vi "Chrg_Dschrg_2.vi"(3 "Strain Offset":dbl, 4 "PS VISA in":refnum<visa-resource-name>, 5 "PS error in":errorcluster caption="PS error in (no error)", 6 "CyclePath":path=path "C:/Users/ga11/Desktop/VI/results/3PtestCharge.lvm" caption="Filename", 7 "Battery Type":T1(ring), 8 "Charge/discharge":enum8{"Charge", "Discharge"}(ring), 9 "Charge/Discharge Voltage Setpoint":dbl format="%#.6g", 11 "Current Setpoint":dbl format="%#.6g", 13 "Current Cutoff":dbl) -> (14 "PS VISA out":refnum<visa-resource-name>, 19 "PS error out":errorcluster)   [LabVIEW 2020]
uses:
  <vilib>/Utility/TradDaqScaling.llb/Convert Strain Gauge Reading (scaler).vi
  stop button2.vi
  Drivers-IT-M3400/IT-M3400.lvlib
panel:
  out "Read Current(A)":dbl format="%.2g"
  out "Read Voltage(V)":dbl format="%.2g"
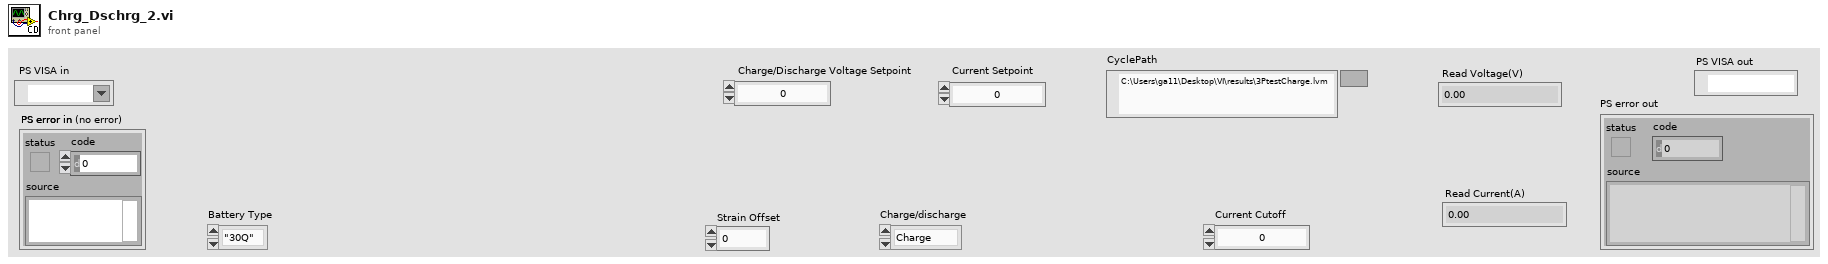
[diagram p1: front panel]
types:
  T1 = enum16{"\"30Q\"", "\"40T\"", "\"2P30Q\"", "\"3P30Q\"", "\"Nissan Leaf\""}
  T2 = cluster{"Baud Rate":u32, "Parity":u16, "Data Bits":u16, "Stop Bits":u16, "Flow Control":u16}
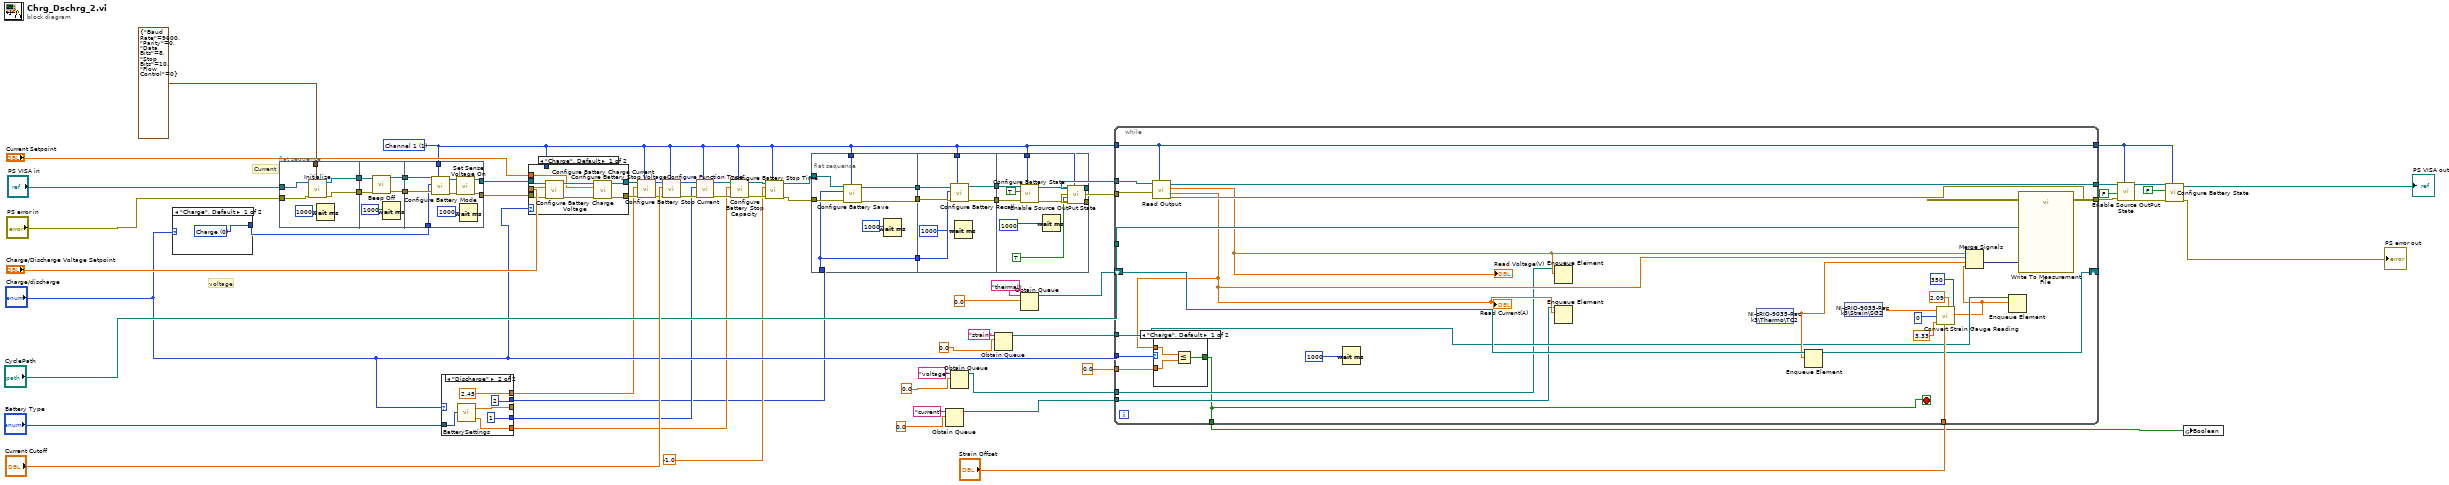
[diagram p0: block diagram]
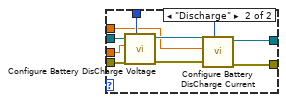
[diagram p2: hidden frame]
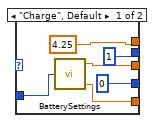
[diagram p3: hidden frame]
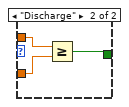
[diagram p4: hidden frame]
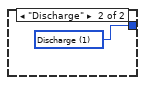
[diagram p5: hidden frame]
diagram:
  w21 = 1 items=["Channel 1"=1, "Channel 2"=2, "Channel 3"=3, "Channel 4"=4, "Channel 5"=5, "Channel 6"=6, "Channel 7"=7, "Channel 8"=8, "Channel 8"=9, "Channel 10"=10, "Channel 11"=11, "Channel 12"=12, "Channel 13"=13, "Channel 14"=14, "Channel 15"=15, "Channel 16"=16] ("Channel")
  # "voltage"
  # "Current"
  n1 = case shown="\"Charge\", Default" "Charge/discharge" {
    tunnel: [w66 w67] -> w29
    frame "Charge", Default {
      w66 = u8 0 items=["Charge", "Discharge"] ("Battery Mode")
    }
    frame "Discharge" {
      w67 = u8 1 items=["Charge", "Discharge"] ("Battery Mode")
    }
  }
  n2 = flat-sequence {
    tunnel: [w69] -> w2
    tunnel: T2 {"Baud Rate"=9600, "Parity"=0, "Data Bits"=8, "Stop Bits"=10, "Flow Control"=0} ("Serial Configuration") -> [w73]
    tunnel: "PS error in" -> [w72]
    tunnel: "PS VISA in" -> [w71]
    tunnel: [w68] -> w1
    tunnel: [w78] -> w50
    tunnel: [w77] -> w49
    tunnel: w2 -> [w76]
    tunnel: w1 -> [w75]
    tunnel: w50 -> [w84]
    tunnel: w49 -> [w86]
    tunnel: w21 -> [w87]
    tunnel: w29 -> [w85]
    tunnel: [w79] -> w18
    tunnel: [w80] -> w17
    frame #0 {
      n3 = call "Initialize.vi"("Serial Configuration"=w73, "error in"=w72, "VISA resource name"=w71) -> ("error out"=w68:errorcluster, "VISA resource name out"=w69:refnum<visa-resource-name>)  [unwired: 7 in]
      n4 = Wait (ms)(milliseconds to wait=1000) -> ()  [unwired: 1 out]
    }
    frame #1 {
      n5 = call "Beep Off.vi"("error in"=w75, "VISA resource name"=w76) -> ("error out"=w77:errorcluster, "VISA resource name out"=w78:refnum<visa-resource-name>)  [unwired: 8 in]
      n6 = Wait (ms)(milliseconds to wait=1000) -> ()  [unwired: 1 out]
    }
    frame #2 {
      n7 = call "Configure Battery Mode.vi"("Channel"=w87, "error in"=w86, "Battery Mode"=w85, "VISA resource name"=w84) -> ("error out"=w81:errorcluster, "VISA resource name out"=w82:refnum<visa-resource-name>)  [unwired: 6 in]
      n8 = call "Set Sense Voltage On.vi"("error in"=w81, "VISA resource name"=w82) -> ("error out"=w79:errorcluster, "VISA resource name out"=w80:refnum<visa-resource-name>)  [unwired: 8 in]
      n9 = Wait (ms)(milliseconds to wait=1000) -> ()  [unwired: 1 out]
    }
  }
  n10 = case shown="\"Discharge\"" "Charge/discharge" {
    tunnel: "Battery Type" -> [w93 w99]
    tunnel: [w92 w97] -> _
    tunnel: [u8 0 ("File") u8 1 ("File")] -> w23
    tunnel: [u8 1 ("File") u8 2 ("File")] -> w20
    tunnel: [w89 w95] -> w22
    tunnel: [4.25 2.45] -> w19
    frame "Charge", Default {
      n11 = call "BatterySettings.vi"("Battery Type"=w93) -> ("RatedCapacity (Ah)"=w89:dbl, "Max Voltage (V)"=w92:dbl)  [unwired: 2 in, 1 out]
    }
    frame "Discharge" {
      n12 = call "BatterySettings.vi"("Battery Type"=w99) -> ("RatedCapacity (Ah)"=w95:dbl, "Min Voltage (V)"=w97:dbl)  [unwired: 2 in, 1 out]
    }
  }
  n13 = case shown="\"Charge\", Default" "Charge/discharge" {
    tunnel: w17 -> [w107 w116]
    tunnel: w18 -> [w106 w115]
    tunnel: [w101 w112] -> w40
    tunnel: [w100 w111] -> w39
    tunnel: w21 -> [_ w110]
    tunnel: "Charge/Discharge Voltage Setpoint" -> [w103 w109]
    tunnel: "Current Setpoint" -> [w102 w108]
    frame "Charge", Default {
      n14 = call "Configure Battery Charge Voltage.vi"("error in"=w106, "Charge Voltage(V)"=w103, "VISA resource name"=w107) -> ("error out"=w104:errorcluster, "VISA resource name out"=w105:refnum<visa-resource-name>)  [unwired: 6 in]
      n15 = call "Configure Battery Charge Current.vi"("error in"=w104, "Charge Current(A)"=w102, "VISA resource name"=w105) -> ("error out"=w100:errorcluster, "VISA resource name out"=w101:refnum<visa-resource-name>)  [unwired: 7 in]
    }
    frame "Discharge" {
      n16 = call "Configure Battery DisCharge Voltage.vi"("Channel"=w110, "error in"=w115, "Discharge Voltage(V)"=w109, "VISA resource name"=w116) -> ("error out"=w113:errorcluster, "VISA resource name out"=w114:refnum<visa-resource-name>)  [unwired: 6 in]
      n17 = call "Configure Battery DisCharge Current.vi"("Channel"=w110, "error in"=w113, "Discharge Current(A)"=w108, "VISA resource name"=w114) -> ("error out"=w111:errorcluster, "VISA resource name out"=w112:refnum<visa-resource-name>)  [unwired: 6 in]
    }
  }
  n18 = call "Configure Battery Stop Voltage.vi"("Channel"=w21, "error in"=w39, "Stop Voltage(V)"=w19, "VISA resource name"=w40) -> ("error out"=w47:errorcluster, "VISA resource name out"=w48:refnum<visa-resource-name>)  [unwired: 6 in]
  n19 = call "Configure Battery Stop Current.vi"("Channel"=w21, "error in"=w47, "Stop Current(A)"="Current Cutoff", "VISA resource name"=w48) -> ("error out"=w25:errorcluster, "VISA resource name out"=w27:refnum<visa-resource-name>)  [unwired: 6 in]
  n20 = call "Configure Function Type.vi"("Channel"=w21, "error in"=w25, "Function Type"=w23, "VISA resource name"=w27) -> ("error out"=w24:errorcluster, "VISA resource name out"=w26:refnum<visa-resource-name>)  [unwired: 6 in]
  n21 = call "Configure Battery Stop Capacity.vi"("Channel"=w21, "error in"=w24, "Stop Capacity(Ah)"=w22, "VISA resource name"=w26) -> ("error out"=w45:errorcluster, "VISA resource name out"=w46:refnum<visa-resource-name>)  [unwired: 6 in]
  n22 = call "Configure Battery Stop Time.vi"("Channel"=w21, "error in"=w45, "Stop Time(S)"=-1.0, "VISA resource name"=w46) -> ("error out"=w31:errorcluster, "VISA resource name out"=w30:refnum<visa-resource-name>)  [unwired: 6 in]
  n23 = flat-sequence {
    tunnel: w20 -> [w122]
    tunnel: w21 -> [w117]
    tunnel: [w120] -> w55
    tunnel: [w122] -> w54
    tunnel: [w119] -> w53
    tunnel: w31 -> [w123]
    tunnel: w30 -> [w121]
    tunnel: [w126] -> w52
    tunnel: [w127] -> w51
    tunnel: w55 -> [w130]
    tunnel: w54 -> [w129]
    tunnel: w53 -> [w128]
    tunnel: w21 -> [w124]
    tunnel: [w134] -> w38
    tunnel: [w133] -> w37
    tunnel: w21 -> [w132]
    tunnel: w52 -> [w140]
    tunnel: w51 -> [w139]
    frame #0 {
      n24 = call "Configure Battery Save.vi"("Channel"=w117, "error in"=w123, "File"=w122, "VISA resource name"=w121) -> ("error out"=w120:errorcluster, "VISA resource name out"=w119:refnum<visa-resource-name>)  [unwired: 6 in]
      n25 = Wait (ms)(milliseconds to wait=1000) -> ()  [unwired: 1 out]
    }
    frame #1 {
      n26 = call "Configure Battery Recall.vi"("Channel"=w124, "error in"=w130, "File"=w129, "VISA resource name"=w128) -> ("error out"=w127:errorcluster, "VISA resource name out"=w126:refnum<visa-resource-name>)  [unwired: 6 in]
      n27 = Wait (ms)(milliseconds to wait=1000) -> ()  [unwired: 1 out]
    }
    frame #2 {
      n28 = call "Configure Battery State.vi"("Channel"=w132, "error in"=w139, "State"=TRUE, "VISA resource name"=w140) -> ("error out"=w137:errorcluster, "VISA resource name out"=w138:refnum<visa-resource-name>)  [unwired: 6 in]
      n29 = Wait (ms)(milliseconds to wait=1000) -> ()  [unwired: 1 out]
      n30 = call "Enable Source OutPut State.vi"("Channel"=w132, "error in"=w137, "State"=TRUE ("Enable Output|Intput"), "VISA resource name"=w138) -> ("error out"=w133:errorcluster, "VISA resource name out"=w134:refnum<visa-resource-name>)  [unwired: 6 in]
    }
  }
  n31 = Obtain Queue(name (unnamed)="current", element data type=0.0) -> (queue out=w8:refnum<queue>)  [unwired: 3 in, 2 out]
  n32 = Obtain Queue(name (unnamed)="voltage", element data type=0.0) -> (queue out=w9:refnum<queue>)  [unwired: 3 in, 2 out]
  n33 = Obtain Queue(name (unnamed)="strain", element data type=0.0) -> (queue out=w12:refnum<queue>)  [unwired: 3 in, 2 out]
  n34 = Obtain Queue(name (unnamed)="thermal", element data type=0.0) -> (queue out=w14:refnum<queue>)  [unwired: 3 in, 2 out]
  n35 = while {
    tunnel: [w159] -> w36
    tunnel: [w157] -> w35
    tunnel: w38 -> [w166]
    tunnel: w37 -> [w165]
    tunnel: w21 -> [w158]
    tunnel: [w158] -> w34
    tunnel: "CyclePath" -> [w163]
    tunnel: 0.0 -> [w161]
    tunnel: "Charge/discharge" -> [w160]
    tunnel: "Strain Offset" -> [w152]
    shift-right: [w149] -> _
    shift-left: w14 -> [w151]
    tunnel: w12 -> [w148]
    tunnel: w9 -> [w144]
    tunnel: w8 -> [w143]
    tunnel: [w141] -> w3
    stop <- w141 stop-if-true
    n36 = call "Read Output.vi"("Channel"=w158, "error in"=w165, "VISA resource name"=w166) -> ("error out"=w157:errorcluster, "Read Current(A)"=w145:dbl, "Read Voltage(V)"=w146:dbl, "VISA resource name out"=w159:refnum<visa-resource-name>)  [unwired: 5 in]
    "Read Voltage(V)" <- w146
    "Read Current(A)" <- w145
    n37 = case shown="\"Charge\", Default" w160 {
      tunnel: w161 -> [w168 w171]
      tunnel: w145 -> [w169 w172]
      tunnel: [w167 w170] -> w141
      frame "Charge", Default {
        n38 = Less Or Equal?(x=w169, y=w168) -> (x <= y?=w167:bool)
      }
      frame "Discharge" {
        n39 = Greater Or Equal?(x=w172, y=w171) -> (x >= y?=w170:bool)
      }
    }
    n40 = Wait (ms)(milliseconds to wait=1000) -> ()  [unwired: 1 out]
    n41 = Enqueue Element(queue=w143, element=w145) -> ()  [unwired: 2 in, 3 out]
    n42 = Enqueue Element(queue=w144, element=w146) -> ()  [unwired: 2 in, 3 out]
    n43 = shared-variable "NI-cRIO-9035-Rack3\\Thermo\\TC2"() -> (w150:dbl)  [unwired: 1 in, 1 out]
    n44 = Enqueue Element(queue=w151, element=w150) -> (queue out=w149:refnum<queue>)  [unwired: 2 in, 2 out]
    n45 = shared-variable "NI-cRIO-9035-Rack3\\Strain\\SG2"() -> (w147:dbl)  [unwired: 1 in, 1 out]
    n46 = call-poly <vilib>:"Convert Strain Gauge Reading.vi"("Vsg (0.0)"=w147, "Bridge Configuration\n(3:Half Bridge II)"=0, "Vex (3.33)"=3.33, "Vinit (0.0)"=w152, "GF (2.0)"=2.09, "Rg (120)"=350) -> ("Strain"=w142:sgl)  [unwired: 4 in]
    n47 = Merge Signals "Merge Signals"(w146, w145, w150, w142) -> (w164:dynamicdata)
    n48 = Enqueue Element(queue=w148, element=w142) -> ()  [unwired: 2 in, 3 out]
    n49 = call "Write To Measurement File"("Signals"=w164, "Filename"=w163) -> ()  [unwired: 15 in, 3 out]
  }
  n50 = call "Enable Source OutPut State.vi"("Channel"=w34, "error in"=w35, "State"=FALSE, "VISA resource name"=w36) -> ("error out"=w43:errorcluster, "VISA resource name out"=w44:refnum<visa-resource-name>)  [unwired: 6 in]
  n51 = call "Configure Battery State.vi"("Channel"=w34, "error in"=w43, "State"=FALSE, "VISA resource name"=w44) -> ("error out"=→"PS error out":errorcluster, "VISA resource name out"=→"PS VISA out":refnum<visa-resource-name>)  [unwired: 6 in]
  n52 = global write "stop button2.vi" "Boolean"(w3) -> ()
